vi "XY Graph With Buffer(Chart).vi"() -> ()   [LabVIEW 2012]
uses:
  <vilib>/Platform/TimedLoop/XDataNode/timing_clust.ctl
  <vilib>/Platform/TimedLoop/XDataNode/nitl_modes.ctl
  <vilib>/Platform/TimedLoop/XDataNode/wakeup.ctl
  <vilib>/Platform/TimedLoop/XDataNode/XDataNode.xnode
  <vilib>/Platform/TimedLoop/XDataNode/XDNodeRunTimeDep.lvlib
panel:
  out "Reverse":T1(graph)
  in  "停止":bool
  out "Random":T1(graph)
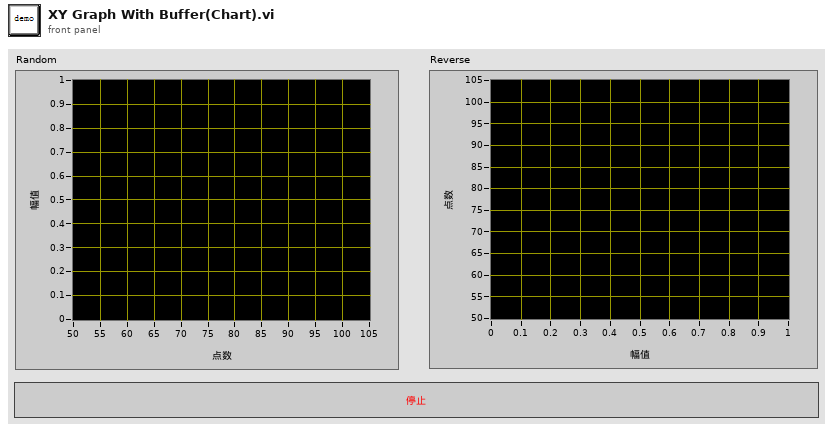
[diagram p1: front panel]
types:
  T1 = cluster{"Current Elements":dbl[], "Current Elements":dbl[]}
  T2 = typedef "XDNodeRunTimeDep.lvlib/timing_clust.ctl" = cluster{"Expected End [f-1]":u64, "Actual End [f-1]":u64, "Finished Late? [f-1]":bool, "Expected End [i-1]":u64, "Actual End [i-1]":u64, "Finished Late? [i-1]":bool, "Expected Start [i]":u64, "Actual Start [i]":u64, "Expected Start [f]":u64, "Actual Start [f]":u64, "Source Name":string, "Structure Name":string, "Period":i64, "Deadline":i64, "Offset":i64, "Start":i64, "Priority":i32, "Timeout":i32, "Mode":T3, "Wakeup Reason":T4, "Error":errorcluster, "Source Type":string, "Secondary Source Type":string, "Global End Time":u64, "Global Start Time":u64, "Frame Duration":u64, "Iteration Duration":u64, "Assigned CPU":i32, "I/O Scan Engine Mode":u32}
  T3 = typedef "XDNodeRunTimeDep.lvlib/nitl_modes.ctl" = enum32{"No Change", "Process missed periods, maintain original phase", "Discard missed periods, maintain original phase", "Process missed periods, ignore original phase", "Discard missed periods, ignore original phase"}
  T4 = typedef "XDNodeRunTimeDep.lvlib/wakeup.ctl" = enum32{"Normal", "Aborted", "Asynchronous wakeup", "Timing source error", "Timed loop error", "Timeout"}
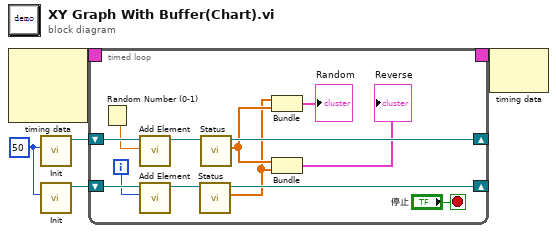
[diagram p0: block diagram]
diagram:
  w1 = 50 ("size")
  n1 = node-c288() -> (w5:T2)  [unwired: 3 in]
  n2 = call "Init.vi"("size"=w1) -> ("FIFO(DBL) 输出"=w3:refnum<class "FIFO(DBL).lvclass">)  [unwired: 9 in, 1 out]
  n3 = call "Init.vi"("size"=w1) -> ("FIFO(DBL) 输出"=w2:refnum<class "FIFO(DBL).lvclass">)  [unwired: 9 in, 1 out]
  n4 = timed-loop {
    timing: w5 -> [_]
    timing-out: [_] -> w4
    shift-right: [w13] -> _
    shift-left: w3 -> [w18]
    shift-right: [w11] -> _
    shift-left: w2 -> [w17]
    i -> [w16]
    stop <- "停止" stop-if-true
    n5 = Random Number (0-1)() -> (number: 0 to 1=w15:dbl)
    n6 = call "Add Element.vi"("Element"=w15, "FIFO(DBL) 输入"=w18) -> ("FIFO(DBL) 输出"=w14:refnum<class "FIFO(DBL).lvclass">)  [unwired: 7 in, 2 out]
    n7 = call "Add Element.vi"("Element"=w16, "FIFO(DBL) 输入"=w17) -> ("FIFO(DBL) 输出"=w12:refnum<class "FIFO(DBL).lvclass">)  [unwired: 7 in, 2 out]
    n8 = call "Status.vi"("FIFO(DBL) 输入"=w12) -> ("Current Elements"=w7:dbl[], "FIFO(DBL) 输出"=w11:refnum<class "FIFO(DBL).lvclass">)  [unwired: 7 in, 2 out]
    n9 = call "Status.vi"("FIFO(DBL) 输入"=w14) -> ("Current Elements"=w8:dbl[], "FIFO(DBL) 输出"=w13:refnum<class "FIFO(DBL).lvclass">)  [unwired: 7 in, 2 out]
    n10 = Bundle("Current Elements"=w7, "Current Elements"=w8) -> (→"Random":T1)  [unwired: 1 in]
    n11 = Bundle("Current Elements"=w8, "Current Elements"=w7) -> (→"Reverse":T1)  [unwired: 1 in]
  }
  n12 = node-c288(w4) -> ()  [unwired: 1 out]
